vi "Kicker Pull Back Routine.vi"(0 "Puck Energy Requirement (mJ)":dbl, 1 "Angle Tolerance (°)":dbl=0.5 format="%#_13g", 4 "stop":bool, 5 "error in (no error)":errorcluster) -> (16 "Kicker Lift Angle (°)":dbl, 17 "Puck Output Velocity (m/s)":dbl, 19 "error out":errorcluster)   [LabVIEW 2017]
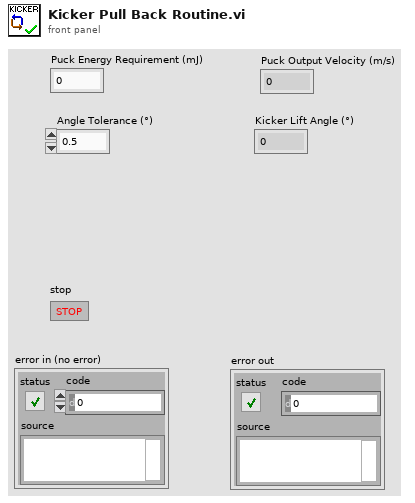
[diagram p1: front panel]
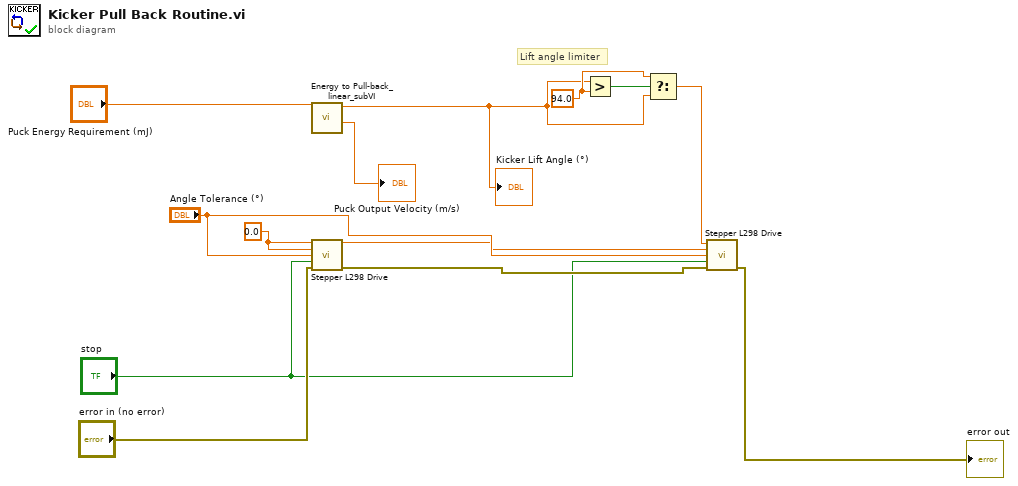
[diagram p0: block diagram]
diagram:
  w3 = 94.0 ("y")
  w10 = 0.0 ("Target Angle (°)")
  # "Lift angle limiter"
  n1 = call "Energy to Pull-back_linear_subVI.vi"("Puck Energy Requirement (mJ)"="Puck Energy Requirement (mJ)") -> ("Output Velocity"=→"Puck Output Velocity (m/s)":dbl, "Pull-back angle (°)"=w2:dbl)  [unwired: 8 in, 1 out]
  "Kicker Lift Angle (°)" <- w2
  n2 = call "Stepper L298 Drive.vi"("Target Angle (0to90)"=w10, "Start Location Step (0to3)"=w10, "Angle Tolerance (°)"="Angle Tolerance (°)", "stop"="stop", "error in (no error)"="error in (no error)") -> ("Current Motor Step (0to3)"=w5:dbl, "error out"=w9:errorcluster)  [unwired: 9 in]
  n3 = Greater?(x=w2, y=w3) -> (0:w4:bool)
  n4 = Select(t=w3, s=w4, f=w2) -> (s? t:f=w1:dbl)
  n5 = call "Stepper L298 Drive.vi"("Target Angle (0to90)"=w1, "Start Location Step (0to3)"=w5, "Angle Tolerance (°)"="Angle Tolerance (°)", "stop"="stop", "error in (no error)"=w9) -> ("error out"=→"error out":errorcluster)  [unwired: 9 in, 1 out]
